vi "Set Websocket Client Handler.vi"(7 "Websocket Client Handler":refnum<class "Websocket Client Handler.lvclass">, 8 "error in (no error)":errorcluster, 11 "Websocket Server in":refnum<class "Websocket Server.lvclass">) -> (0 "error out":errorcluster, 3 "Websocket Server out":refnum<class "Websocket Server.lvclass">)   [LabVIEW 2016, in "Stream Mediator.lvlib" / "Websocket Server.lvclass"]
doc: "--\nCopyright © 2017 Composed SystemsI All rights reserved.\n\nAuthor: Jon McBee <jon.mcbee@composed.io>\n\nThis library is provided \"AS IS\" ,WITHOUT WARRANTIES OR\nCONDITIONS OF ANY KIND, either express or implied.\n\nComposed Systems -- composed.io\n\nStream 0.0.1.1\nJon McBee - Composed Systems\nCopyright (c) 2017, Composed Systems"
uses:
  <userlib>/Composed Systems/Stream/Mediator/Classes/Websocket Server Actor/Websocket Server/Websocket Server.lvclass
  <userlib>/Composed Systems/Stream/Mediator/Classes/Websocket Client Handler Actor/Websocket Client Handler/Websocket Client Handler.lvclass
  <userlib>/Composed Systems/Stream/Mediator/Classes/Websocket Server Actor/Websocket Server/Websocket Server.lvclass/Websocket Server.ctl
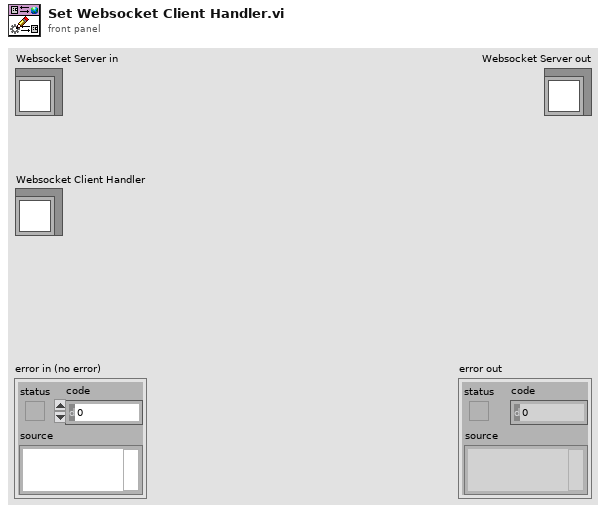
[diagram p1: front panel]
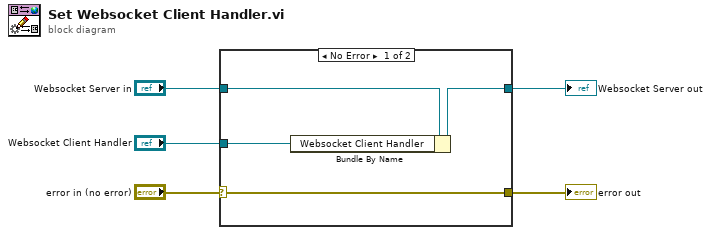
[diagram p0: block diagram]
diagram:
  n1 = case shown="No Error" "error in (no error)" {
    selector: "error in (no error)" -> [w9 w11]
    tunnel: [w9 w11] -> w4
    tunnel: [w7 w10] -> w2
    tunnel: "Websocket Server in" -> [w8 w10]
    tunnel: "Websocket Client Handler" -> [w6 _]
    frame No Error {
      n2 = Bundle By Name(cluster=w8, "Websocket Client Handler"=w6) -> (w7:refnum<class "Websocket Server.lvclass">)
    }
    frame Error {
    }
  }
  "error out" <- w4
  "Websocket Server out" <- w2
